vi "Encoded UTF-8 String to Encoded UTF-16LE String.vi"(9 "error in":errorcluster, 10 "Encoded UTF-8 String":T2) -> (1 "error out":errorcluster, 2 "Encoded UTF-16LE String":T1)   [LabVIEW 2020, in "G-Unicode.lvlib"]
uses:
  G-Unicode.lvlib
  Types/Encoded UTF-8 String.ctl
  Types/Encoded UTF-16LE String.ctl
  lib/g_unicode_32.dll
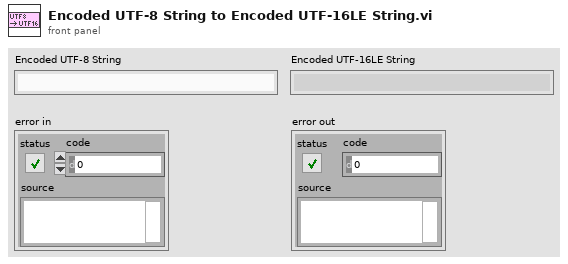
[diagram p1: front panel]
types:
  T1 = typedef "G-Unicode.lvlib/Encoded UTF-16LE String.ctl" = string
  T2 = typedef "G-Unicode.lvlib/Encoded UTF-8 String.ctl" = string
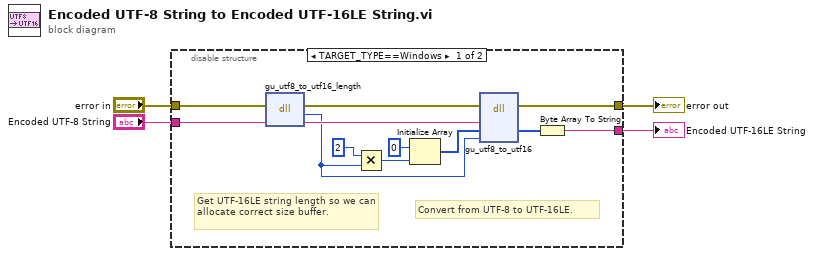
[diagram p0: block diagram]
diagram:
  n1 = disable-structure shown="TARGET_TYPE==Windows" {
    disable-tunnel: "Encoded UTF-8 String" -> [w16 w17]
    disable-tunnel: [w9 w17] -> w1
    disable-tunnel: "error in" -> [w6 w18]
    disable-tunnel: [w8 w18] -> w2
    frame condition #0 (active) {
      # "Convert from UTF-8 to UTF-16LE."
      # "Get UTF-16LE string length so we can allocate correct size buffer."
      n2 = dll-call lib="C:/github/dataflowg/g-unicode/src/LabVIEW/G-Unicode/lib/g_unicode_*.*" fn="gu_utf8_to_utf16_length"(error in=w6, "utf8"=w16) -> (error out=w7:errorcluster, "length"=w5:i32, "utf8"=w11:string)  [unwired: 2 in, 1 out]
      n3 = Multiply(x=2 ("y"), y=w5) -> (x*y=w14:i32)
      n4 = Initialize Array(u8 0 ("dwFlags"), w14) -> (w12:u8[])
      n5 = dll-call lib="C:/github/dataflowg/g-unicode/src/LabVIEW/G-Unicode/lib/g_unicode_*.*" fn="gu_utf8_to_utf16"(error in=w7, "utf8"=w11, "urf16le"=w12, "utf16le_length"=w5) -> (error out=w8:errorcluster, "urf16le"=w10:u8[])  [unwired: 5 in, 1 out]
      n6 = Byte Array To String(unsigned byte array=w10) -> (string=w9:string)
    }
    frame condition #1 {
    }
  }
  "error out" <- w2
  "Encoded UTF-16LE String" <- w1
